vi "Write register.vi"(8 "error in (no error)":errorcluster, 9 "Write Data":variant, 10 "Start address":string, 11 "PLCMonitor in":refnum<class "PLCMonitor.lvclass">) -> (0 "error out":errorcluster, 3 "PLCMonitor out":refnum<class "PLCMonitor.lvclass">)   [LabVIEW 2020, in "PLCMonitor.lvlib" / "PLCMonitor.lvclass"]
uses:
  PLCMonitor.lvclass
  PLCMonitor.lvclass/PLCMonitor.ctl
  HslCommunication/Abstract PLC Controler/Abs Controler.lvclass
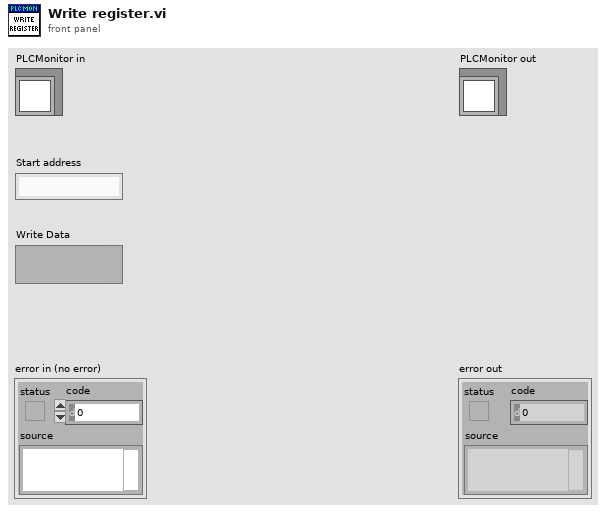
[diagram p1: front panel]
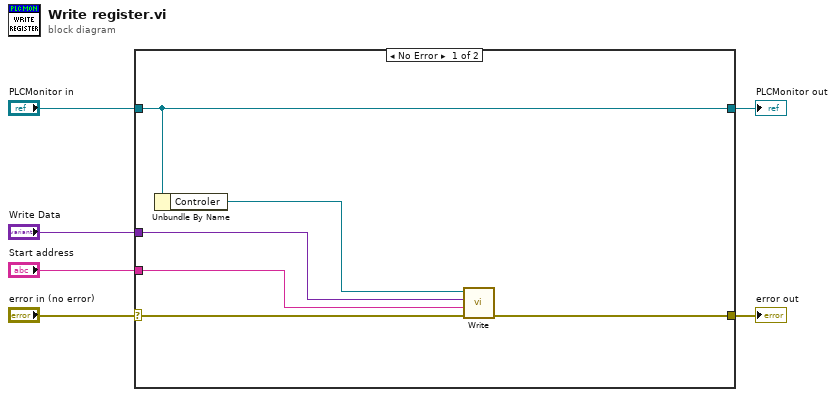
[diagram p0: block diagram]
diagram:
  n1 = case shown="No Error" "error in (no error)" {
    selector: "error in (no error)" -> [w12 w14]
    tunnel: [w11 w14] -> w5
    tunnel: [w10 w13] -> w3
    tunnel: "PLCMonitor in" -> [w10 w13]
    tunnel: "Start address" -> [w8 _]
    tunnel: "Write Data" -> [w7 _]
    frame No Error {
      n2 = Unbundle By Name(w10) -> ("Controler"=w9:refnum<class "Abs Controler.lvclass">)
      n3 = call-dynamic "Write.vi"("error in (no error)"=w12, "Start address"=w8, "Read Type"=w7, "MelsecTCP in"=w9) -> ("error out"=w11:errorcluster)  [unwired: 6 in, 1 out]
    }
    frame Error {
    }
  }
  "error out" <- w5
  "PLCMonitor out" <- w3
